vi "RegisterAssignmentScan.vi"(8 "error in (no error)":errorcluster, 11 "Register Map File":path) -> (0 "error out":errorcluster, 2 "Register Names":string[](array[string]), 3 "RegMap Data":T1[](array[typedef]) {"Address" format="%.0x"; "Base" format="%.0x"})   [LabVIEW 2010]
doc: "This VI read the register map text file and parses the contents. The file data is returned as an array of register names and an array of data cluster.\n\nInputs:\nRegister Map File - path of the register map text file (see block diagram for structure)\nerror in - error input cluster\n\nOutputs:\nRegister Names - (str []) array of controls register names read from the files\nRegMap Data - (cluster[]) array of cluster containing register data from files\n -> Address (int) - address of the control register\n -> Name (str) - name of the register\n -> Base (int) - base value of the register; determined by substituting 0s for functional group characters\n -> Item (cluster[]) - array of cluster containing register function details. Each item in the array represents a separate function (bit(s)).\n -> LSB (int) - LSB of the function in the register\n -> MSB (int) - MSB of the function in the register\n -> Multi? (bool) - TRUE is function is controlled by multiple bits in the register\nerror out - error output cluster"
uses:
  Controls/Shift Registers/TYP_CtrlReg.ctl
  Controls/TYP_CtrlRegItem.ctl
  <vilib>/Utility/file.llb/Read From Spreadsheet File (string).vi
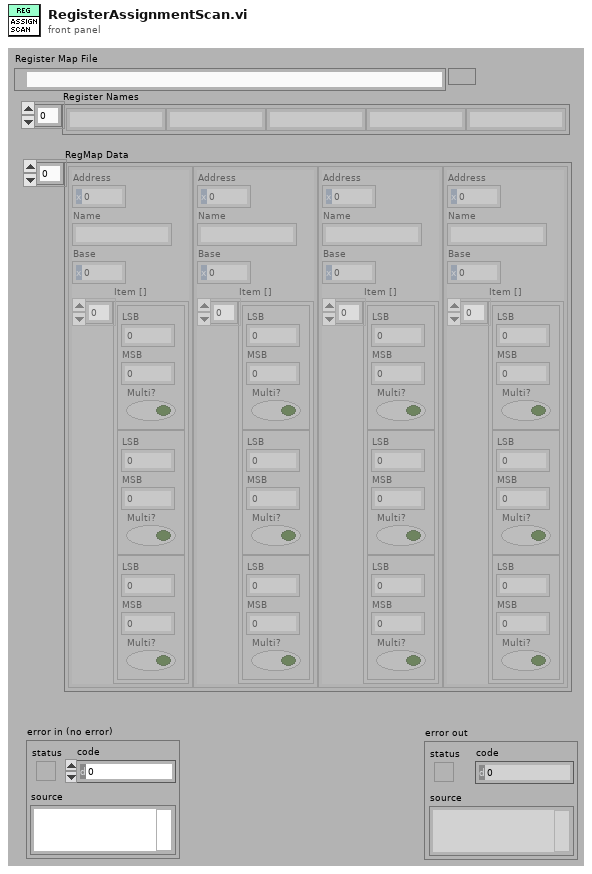
[diagram p1: front panel]
types:
  T1 = typedef "TYP_CtrlReg.ctl" = cluster{"Address":u8, "Name":string, "Base":i8, "Item []":T2[]}
  T2 = typedef "TYP_CtrlRegItem.ctl" = cluster{"LSB":u8, "MSB":u8, "Multi?":bool}
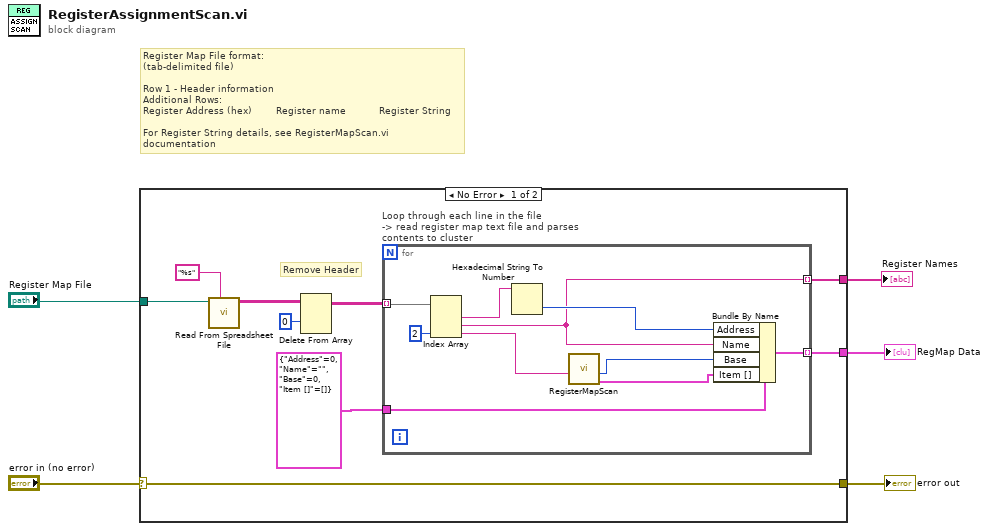
[diagram p0: block diagram]
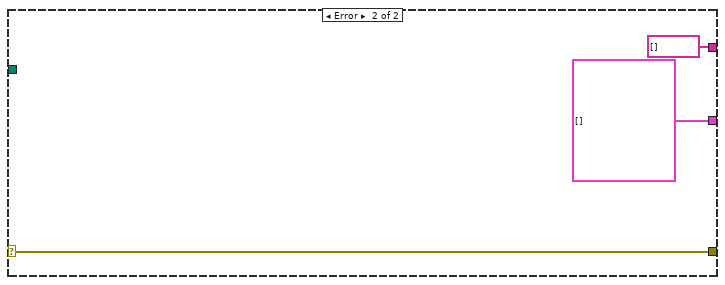
[diagram p2: hidden frame]
diagram:
  # "Register Map File format:\n(tab-delimited file)\n\nRow 1 - Header information\nAdditional Rows:\nRegister Address (hex)        Register name           Register String \n\nFor Register String details, see RegisterMapScan.vi documentation"
  n1 = case shown="No Error" "error in (no error)" {
    selector: "error in (no error)" -> [w7 w27]
    tunnel: "Register Map File" -> [w13 _]
    tunnel: [w11 T1[] []] -> w4
    tunnel: [w7 w27] -> w2
    tunnel: [w6 string[] []] -> w1
    frame No Error {
      # "Remove Header"
      n2 = call-poly <vilib>:"Read From Spreadsheet File.vi"("format (%s)"="%s" ("format (%.3f)"), "file path (dialog if empty)"=w13) -> ("all rows"=w10:string[][])  [unwired: 2 in, 7 out]
      n3 = Delete From Array(array=w10, index (row)=0) -> (array with subset deleted=w8:string[][])  [unwired: 2 in, 1 out]
      n4 = for "Loop through each line in the file\n-> read register map text file and parses contents to cluster" {
        tunnel: w8 -> [w24] mode=indexing
        tunnel: T1 {"Address"=0, "Name"="", "Base"=0, "Item []"=[]} ("CtrlRegister Data") -> [w21]
        tunnel: [w17] -> w11 mode=indexing
        tunnel: [w16] -> w6 mode=indexing
        n5 = Index Array(array=w24, index #3=2 ("index")) -> (element #1=w22:string, element #2=w16:string, element #3=w15:string)  [unwired: 2 in]
        n6 = Hexadecimal String To Number(string=w22) -> (number=w20:u32)  [unwired: 3 out]
        n7 = call "RegisterMapScan.vi"("Register Map"=w15) -> ("Item Array"=w18:T2[], "Base"=w19:u8)  [unwired: 9 out]
        n8 = Bundle By Name(cluster=w21, "Address"=w20, "Name"=w16, "Base"=w19, "Item []"=w18) -> (w17:T1)
      }
    }
    frame Error {
    }
  }
  "RegMap Data" <- w4
  "error out" <- w2
  "Register Names" <- w1
